vi "Catagorize Library.vi"(8 "error in (no error)":errorcluster {"code" format="Error %.0f"}, 10 "Library":refnum<vi>, 11 "VIDoc Parser In":refnum<class "VIDoc Parser.lvclass">) -> (0 "error out":errorcluster {"code" format="Error %.0f"}, 2 "Is Library?":bool, 3 "VIDoc Parser Out":refnum<class "VIDoc Parser.lvclass">)   [LabVIEW 2023, in "VIDoc Parsing.lvlib" / "VIDoc Parser.lvclass"]
uses:
  VIDoc Parser.lvclass
  VIDoc Parser.lvclass/VIDoc Parser.ctl
  Library Documentation/Library Documentation.lvclass
  Interface Documenation/Interface Documenation.lvclass
  Class Documentation/Class Documentation.lvclass
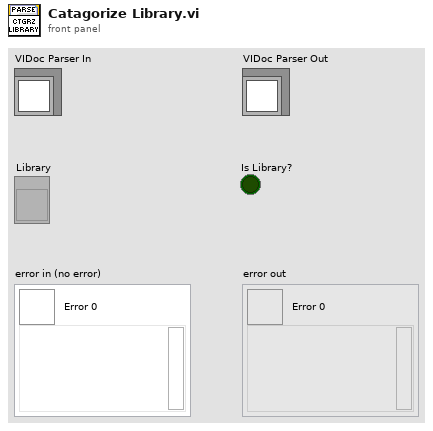
[diagram p1: front panel]
types:
  T1 = typedef "VIDoc Parsing.lvlib/Parser Settings.lvclass/Parser Settings Cluster.ctl" = cluster{"Draw Controls":T2, "Max Control Recursion Depth":i32, "Bookmarks Map":map{string, string[]}}
  T2 = typedef "VIDoc Parsing.lvlib/Parser Settings.lvclass/Draw Controls Cluster.ctl" = cluster{"Subpanels":bool, "Tabs":bool, "TypeDefs":bool, "Error Clusters":T3, "DVRs":T3, "Queues & Notifiers":T3}
  T3 = typedef "VIDoc Parsing.lvlib/Parser Settings.lvclass/Draw Option Enum.ctl" = enum16{"Ignore", "Draw", "Draw + Contents"}
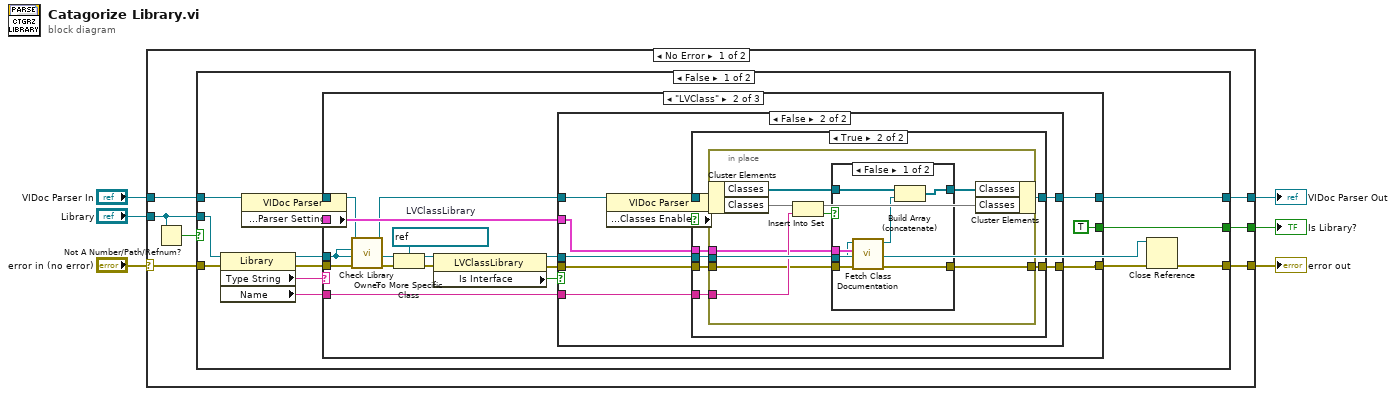
[diagram p0: block diagram]
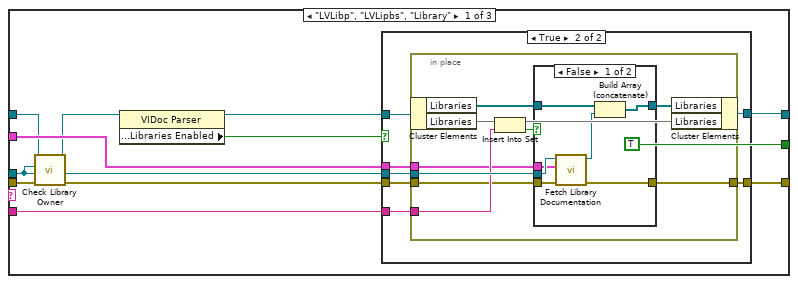
[diagram p2: hidden frame]
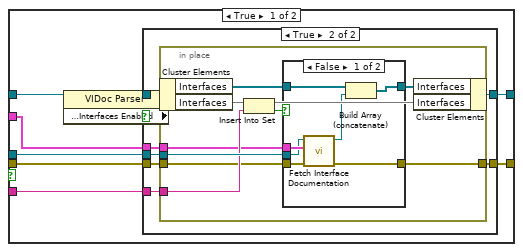
[diagram p5: hidden frame]
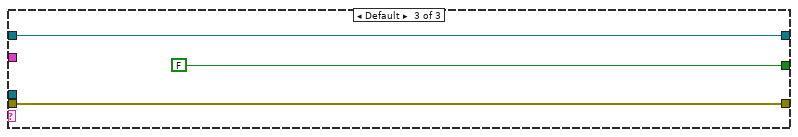
[diagram p10: hidden frame]
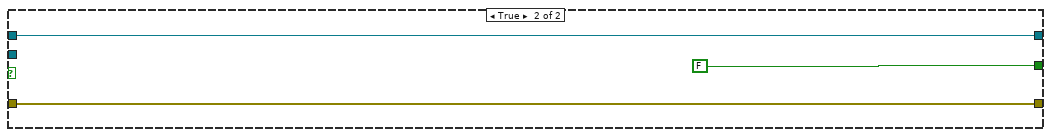
[diagram p11: hidden frame]
diagram:
  n1 = case shown="No Error" "error in (no error)" {
    selector: "error in (no error)" -> [w12 w164]
    tunnel: [w11 w164] -> w5
    tunnel: [w10 w163] -> w3
    tunnel: "VIDoc Parser In" -> [w9 w163]
    tunnel: "Library" -> [w7 _]
    tunnel: [w8 _] -> w1
    frame No Error {
      n2 = Not A Number/Path/Refnum?(number/path/refnum=w7) -> (NaN/Path/Refnum?=w13:bool)
      n3 = case shown="False" w13 {
        tunnel: w12 -> [w25 w162]
        tunnel: [w15 w162] -> w11
        tunnel: [w22 w161] -> w10
        tunnel: w9 -> [w23 w161]
        tunnel: w7 -> [w26 _]
        tunnel: [w21 FALSE] -> w8
        frame False {
          n4 = property class="Library"(reference=w26, error in=w25) -> (reference out=w14:refnum<vi>, error out=w19:errorcluster, "Type String"=w24:string, "Name"=w20:string)
          n5 = property class="VIDoc Parser"(reference=w23) -> (reference out=w17:refnum<class "VIDoc Parser.lvclass">, "Properties:Settings:Parser Settings"=w16:T1)  [unwired: 1 in, 1 out]
          n6 = case shown="\"LVClass\"" w24 {
            tunnel: w17 -> [w29 w73 w159]
            tunnel: [w38 w82 w159] -> w22
            tunnel: w14 -> [w31 w71 _]
            tunnel: [TRUE TRUE FALSE] -> w21
            tunnel: w20 -> [w36 w76 _]
            tunnel: w19 -> [w32 w74 w157]
            tunnel: [w35 w67 w157] -> w18
            tunnel: w16 -> [w34 w75 _]
            frame "LVLibp", "LVLipbs", "Library" {
              n7 = call "Check Library Owner.vi"("Error in"=w32, "Library"=w31, "VIDoc Parser In"=w29) -> ("Error out"=w33:errorcluster, "VIDoc Parser Out"=w30:refnum<class "VIDoc Parser.lvclass">)  [unwired: 7 in]
              n8 = property class="VIDoc Parser"(reference=w30) -> (reference out=w28:refnum<class "VIDoc Parser.lvclass">, "Properties:Enabled:Libraries Enabled"=w27:bool)  [unwired: 1 in, 1 out]
              n9 = case shown="True" w27 {
                tunnel: [w40 w47] -> w38
                tunnel: w36 -> [_ w46]
                tunnel: [w39 w45] -> w35
                tunnel: w34 -> [_ w44]
                tunnel: w33 -> [w39 w43]
                tunnel: w31 -> [_ w42]
                tunnel: w28 -> [w40 w41]
                frame False {
                }
                frame True {
                  n10 = in-place {
                    in-place-border: w42 -> [w56]
                    in-place-border: w46 -> [w53]
                    in-place-border: w43 -> [w50]
                    in-place-border: [w49] -> w45
                    in-place-border: w44 -> [w48]
                    n11 = in-place-cluster #1(w41) -> ("Libraries"=w57:refnum<class "Library Documentation.lvclass">[], "Libraries"=w55:set{string})
                    n12 = Insert Into Set(10:w53, 11:w55) -> (2:w52:bool, 3:w54:set{string})
                    n13 = case shown="False" w52 {
                      tunnel: w57 -> [w64 w66]
                      tunnel: [w63 w66] -> w51
                      tunnel: w56 -> [w59 _]
                      tunnel: w50 -> [w62 w65]
                      tunnel: [w61 w65] -> w49
                      tunnel: w48 -> [w58 _]
                      frame False {
                        n14 = call "Fetch Library Documentation.vi"("error in (no error)"=w62, "Parser Settings"=w58, "Library in"=w59) -> ("error out"=w61:errorcluster, "Library Documentation Out"=w60:refnum<class "Library Documentation.lvclass">)  [unwired: 7 in]
                        n15 = Build Array (concatenate)(w64, w60) -> (w63:refnum<class "Library Documentation.lvclass">[])
                      }
                      frame True {
                      }
                    }
                    n16 = in-place-cluster #1("Libraries"=w51, "Libraries"=w54) -> (w47:refnum<class "VIDoc Parser.lvclass">)
                  }
                }
              }
            }
            frame "LVClass" {
              w81 = refnum<vi> refnum  # LVClassLibrary
              n17 = call "Check Library Owner.vi"("Error in"=w74, "Library"=w71, "VIDoc Parser In"=w73) -> ("Error out"=w70:errorcluster, "VIDoc Parser Out"=w72:refnum<class "VIDoc Parser.lvclass">)  [unwired: 7 in]
              n18 = To More Specific Class(target class=w81, reference=w71, error in=w70) -> (specific class reference=w80:refnum<vi>, error out=w79:errorcluster)
              n19 = property class="LVClassLibrary"(reference=w80, error in=w79) -> (reference out=w68:refnum<vi>, error out=w69:errorcluster, "Is Interface"=w78:bool)
              n20 = case shown="False" w78 {
                tunnel: w72 -> [w91 w128]
                tunnel: [w90 w127] -> w82
                tunnel: w76 -> [w88 w125]
                tunnel: w75 -> [w89 w126]
                tunnel: w69 -> [w87 w124]
                tunnel: w68 -> [w86 w123]
                tunnel: [w85 w122] -> w67
                frame True {
                  n21 = property class="VIDoc Parser"(reference=w91) -> (reference out=w84:refnum<class "VIDoc Parser.lvclass">, "Properties:Enabled:Interfaces Enabled"=w83:bool)  [unwired: 1 in, 1 out]
                  n22 = case shown="True" w83 {
                    tunnel: [w93 w100] -> w90
                    tunnel: w89 -> [_ w99]
                    tunnel: w88 -> [_ w98]
                    tunnel: w87 -> [w92 w97]
                    tunnel: w86 -> [_ w96]
                    tunnel: [w92 w95] -> w85
                    tunnel: w84 -> [w93 w94]
                    frame False {
                    }
                    frame True {
                      n23 = in-place {
                        in-place-border: w96 -> [w109]
                        in-place-border: w98 -> [w106]
                        in-place-border: w97 -> [w103]
                        in-place-border: [w102] -> w95
                        in-place-border: w99 -> [w101]
                        n24 = in-place-cluster #2(w94) -> ("Interfaces"=w110:refnum<class "Interface Documenation.lvclass">[], "Interfaces"=w108:set{string})
                        n25 = Insert Into Set(10:w106, 11:w108) -> (2:w105:bool, 3:w107:set{string})
                        n26 = case shown="False" w105 {
                          tunnel: w110 -> [w117 w119]
                          tunnel: [w116 w119] -> w104
                          tunnel: w109 -> [w111 _]
                          tunnel: w103 -> [w115 w118]
                          tunnel: [w114 w118] -> w102
                          tunnel: w101 -> [w112 _]
                          frame False {
                            n27 = call "Fetch Interface Documentation.vi"("error in (no error)"=w115, "Parser Settings"=w112, "Interface in"=w111) -> ("error out"=w114:errorcluster, "Interface Documenation Out"=w113:refnum<class "Interface Documenation.lvclass">)  [unwired: 7 in]
                            n28 = Build Array (concatenate)(w117, w113) -> (w116:refnum<class "Interface Documenation.lvclass">[])
                          }
                          frame True {
                          }
                        }
                        n29 = in-place-cluster #2("Interfaces"=w104, "Interfaces"=w107) -> (w100:refnum<class "VIDoc Parser.lvclass">)
                      }
                    }
                  }
                }
                frame False {
                  n30 = property class="VIDoc Parser"(reference=w128) -> (reference out=w121:refnum<class "VIDoc Parser.lvclass">, "Properties:Enabled:Classes Enabled"=w120:bool)  [unwired: 1 in, 1 out]
                  n31 = case shown="True" w120 {
                    tunnel: [w130 w137] -> w127
                    tunnel: w126 -> [_ w136]
                    tunnel: w125 -> [_ w135]
                    tunnel: w124 -> [w129 w134]
                    tunnel: w123 -> [_ w133]
                    tunnel: [w129 w132] -> w122
                    tunnel: w121 -> [w130 w131]
                    frame False {
                    }
                    frame True {
                      n32 = in-place {
                        in-place-border: w133 -> [w146]
                        in-place-border: w135 -> [w143]
                        in-place-border: w134 -> [w140]
                        in-place-border: [w139] -> w132
                        in-place-border: w136 -> [w138]
                        n33 = in-place-cluster #3(w131) -> ("Classes"=w147:refnum<class "Class Documentation.lvclass">[], "Classes"=w145:set{string})
                        n34 = Insert Into Set(10:w143, 11:w145) -> (2:w142:bool, 3:w144:set{string})
                        n35 = case shown="False" w142 {
                          tunnel: w147 -> [w154 w156]
                          tunnel: [w153 w156] -> w141
                          tunnel: w146 -> [w148 _]
                          tunnel: w140 -> [w152 w155]
                          tunnel: [w151 w155] -> w139
                          tunnel: w138 -> [w149 _]
                          frame False {
                            n36 = call "Fetch Class Documentation.vi"("error in"=w152, "Parser Settings"=w149, "Class in"=w148) -> ("error out"=w151:errorcluster, "Class Documentation Out"=w150:refnum<class "Class Documentation.lvclass">)  [unwired: 7 in]
                            n37 = Build Array (concatenate)(w154, w150) -> (w153:refnum<class "Class Documentation.lvclass">[])
                          }
                          frame True {
                          }
                        }
                        n38 = in-place-cluster #3("Classes"=w141, "Classes"=w144) -> (w137:refnum<class "VIDoc Parser.lvclass">)
                      }
                    }
                  }
                }
              }
            }
            frame Default {
            }
          }
          n39 = Close Reference(reference=w14, error in (no error)=w18) -> (error out=w15:errorcluster)
        }
        frame True {
        }
      }
    }
    frame Error {
    }
  }
  "error out" <- w5
  "VIDoc Parser Out" <- w3
  "Is Library?" <- w1
